vi "GenerateData.vi"(8 "error in (no error)":errorcluster, 11 "String in":refnum<class "String.lvclass">) -> (0 "error out":errorcluster, 3 "String out":refnum<class "String.lvclass">)   [LabVIEW 2023, in "String.lvclass"]
uses:
  String.lvclass
  C:/Users/santharu.subramanian/Documents/LV New Assignments/Sender-Receiver/Classes/Data/Data.lvclass
  String.lvclass/String.ctl
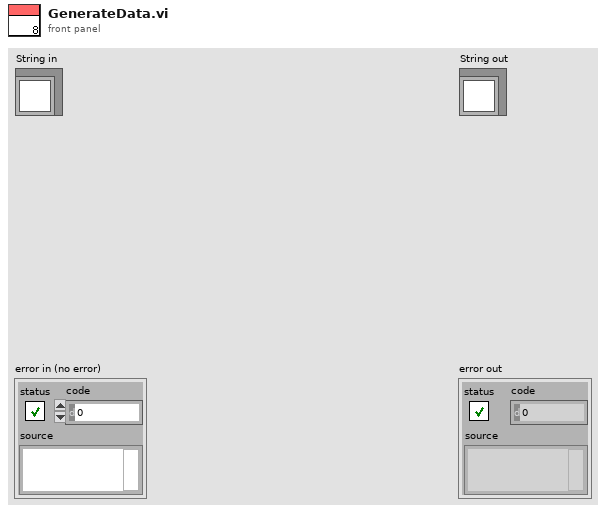
[diagram p1: front panel]
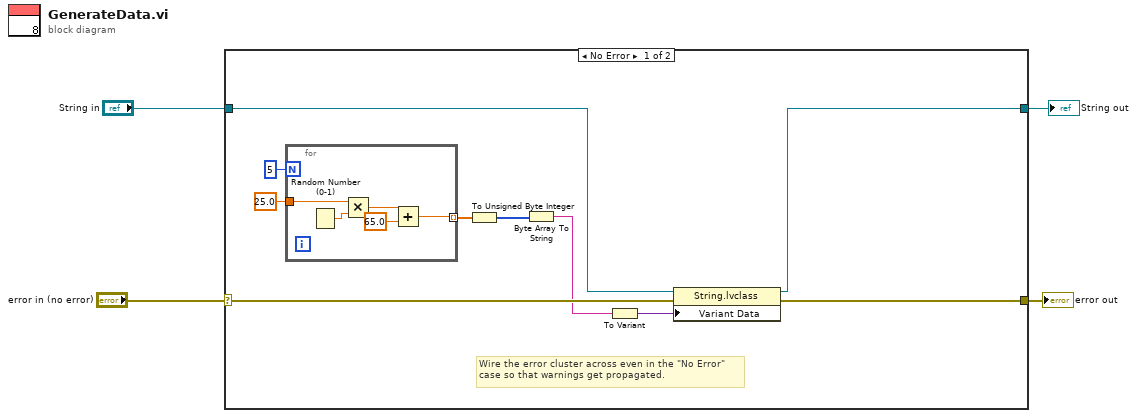
[diagram p0: block diagram]
diagram:
  n1 = case shown="No Error" "error in (no error)" {
    selector: "error in (no error)" -> [w14 w21]
    tunnel: [w13 w21] -> w3
    tunnel: [w11 w20] -> w1
    tunnel: "String in" -> [w12 w20]
    frame No Error {
      # "Wire the error cluster across even in the \"No Error\"\ncase so that warnings get propagated."
      n2 = for {
        N: 5 -> [_]
        tunnel: 25.0 ("x") -> [w19]
        tunnel: [w15] -> w8 mode=indexing
        n3 = Random Number (0-1)() -> (number: 0 to 1=w18:dbl)
        n4 = Multiply(x=w19, y=w18) -> (x*y=w17:dbl)
        n5 = Add(x=w17, y=65.0) -> (x+y=w15:dbl)
      }
      n6 = To Unsigned Byte Integer(number=w8) -> (unsigned 8bit integer=w7:u8[])
      n7 = Byte Array To String(unsigned byte array=w7) -> (string=w6:string)
      n8 = To Variant(anything=w6) -> (Variant=w5:variant)
      n9 = property class="String.lvclass"(reference=w12, error in=w14, "Variant Data"=w5) -> (reference out=w11:refnum<class "String.lvclass">, error out=w13:errorcluster)
    }
    frame Error {
    }
  }
  "error out" <- w3
  "String out" <- w1
